vi "Init.vi"(8 "error in (no error)":errorcluster, 11 "Socket":refnum<k5>) -> (0 "error out":errorcluster, 3 "Request out":refnum<class "Request.lvclass">)   [LabVIEW 2017, in "Request.lvclass"]
uses:
  Request.lvclass
  Request.lvclass/Request.ctl
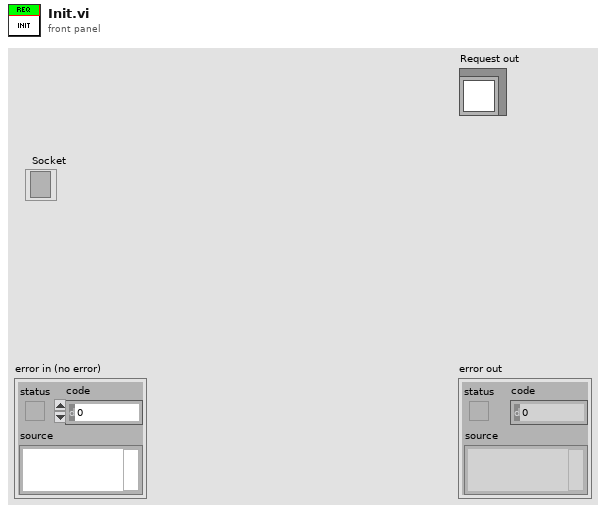
[diagram p1: front panel]
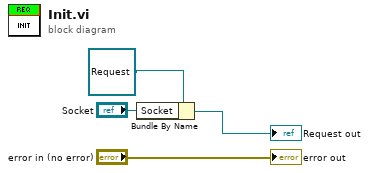
[diagram p0: block diagram]
diagram:
  n1 = Bundle By Name(cluster=refnum<class "Request.lvclass"> refnum ("Request in"), "Socket"="Socket") -> (→"Request out":refnum<class "Request.lvclass">)
  "error out" <- "error in (no error)"
